vi "BodeAnalysis.vi"(8 "error in (no error)":errorcluster, 9 "Reference Ampltide(P2P)":dbl, 10 "Max Frequency":dbl, 11 "FPGA Interface":refnum<k20>) -> (0 "error out":errorcluster)   [LabVIEW 2013]
uses:
  <vilib>/rvi/interface/nirviReadWriteControl/nirviReadWriteControl.xnode
  <vilib>/rvi/interface/Simulation/niFpgaSimulationCallBeginRW.vi
  <vilib>/rvi/errors/niLvFpgaAdjustHostInterfaceError.vi
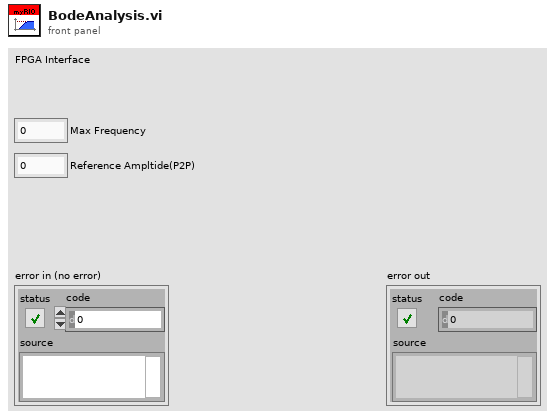
[diagram p1: front panel]
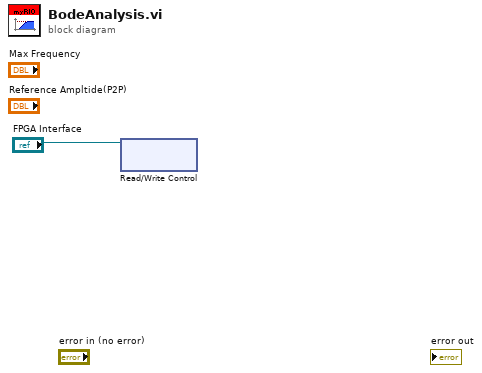
[diagram p0: block diagram]
diagram:
  n1 = xnode "Read/Write Control"("FPGA VI Reference In"="FPGA Interface") -> ()  [unwired: 1 in, 3 out]
